vi "Update_msg_B2.vi"(8 "error in (no error)":errorcluster, 10 "Status":string, 11 "Button_transfer in":refnum<class "Button_transfer.lvclass">) -> (0 "error out":errorcluster, 3 "Button_transfer out":refnum<class "Button_transfer.lvclass">)   [LabVIEW 2025, in "Button_transfer.lvlib" / "Button_transfer.lvclass"]
uses:
  Button_transfer.lvclass
  Button_transfer.lvclass/Button_transfer.ctl
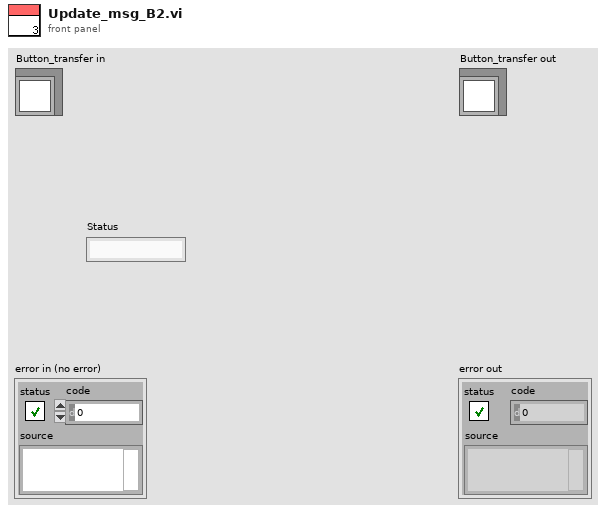
[diagram p1: front panel]
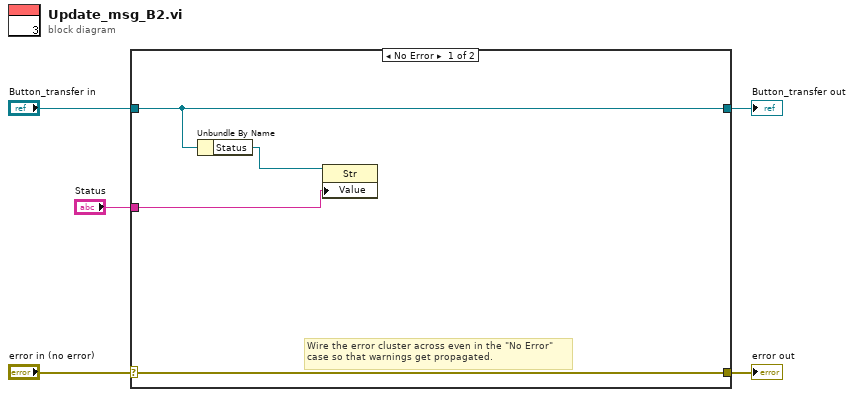
[diagram p0: block diagram]
diagram:
  n1 = case shown="No Error" "error in (no error)" {
    selector: "error in (no error)" -> [w9 w11]
    tunnel: [w9 w11] -> w4
    tunnel: [w8 w10] -> w2
    tunnel: "Button_transfer in" -> [w8 w10]
    tunnel: "Status" -> [w6 _]
    frame No Error {
      # "Wire the error cluster across even in the \"No Error\"\ncase so that warnings get propagated."
      n2 = Unbundle By Name(w8) -> ("Status"=w7:refnum<vi>)
      n3 = property class="Str"(reference=w7, "Value"=w6) -> ()  [unwired: 1 in, 2 out]
    }
    frame Error {
    }
  }
  "error out" <- w4
  "Button_transfer out" <- w2
